vi "ziZoomFFT-SNR.vi"(7 "window properties":cluster{"eq noise BW":dbl, "coherent gain":dbl}={"eq noise BW"=1.0, "coherent gain"=1.0} {"coherent gain" format="%0.2f"; "eq noise BW" format="%0.2f"}, 8 "Order (#)":i32=8, 9 "Timeconstant (s)":dbl format="%#_3p", 10 "Powerspectrum (Vrms^2)":dbl[](array[numeric]), 11 "Freqs (Hz)":dbl[](array[numeric])) -> (0 "Segmentation":cluster{"Freqs (Hz)":dbl[], dbl[]}[](array[cluster]), 1 "Noise BW (Hz)":dbl format="%_3g", 2 "Noise (Vrms^2)":dbl format="%_3g", 3 "Signal BW (Hz)":dbl format="%_3g", 4 "Noise PSD (Vrms/rtHz)":dbl format="%_6p", 5 "Signal (Vrms^2)":dbl format="%_3p", 6 "Peak PSD (Vrms/rtHz)":dbl format="%_6p")   [LabVIEW 2009, in "Zurich Instruments LabOne.lvlib"]
doc: "Calculates:\n\nSNR = \"power in signal band\" / \"power in noise band\"\n\nThe Segmentation output contains an array with:\n\n0: Signal band\n1: Fitted noise\n2: Lower noise band\n3: Upper noise band"
uses:
  <instrlib>/Zurich Instruments LabOne/Zurich Instruments LabOne.lvlib
panel:
  out "Noise Level (Vrms^2)":dbl format="%_6p"
  out "Spectral SNR":dbl format="%_3p"
  out "Segmentation Plot":cluster{"Y":dbl[], "Y":dbl[]}[](graph)
  out "val-trans":dbl[](graph)
  out "Spectral Peak - Noise Separation":dbl format="%_6p"
  out "sorted":dbl[](graph)
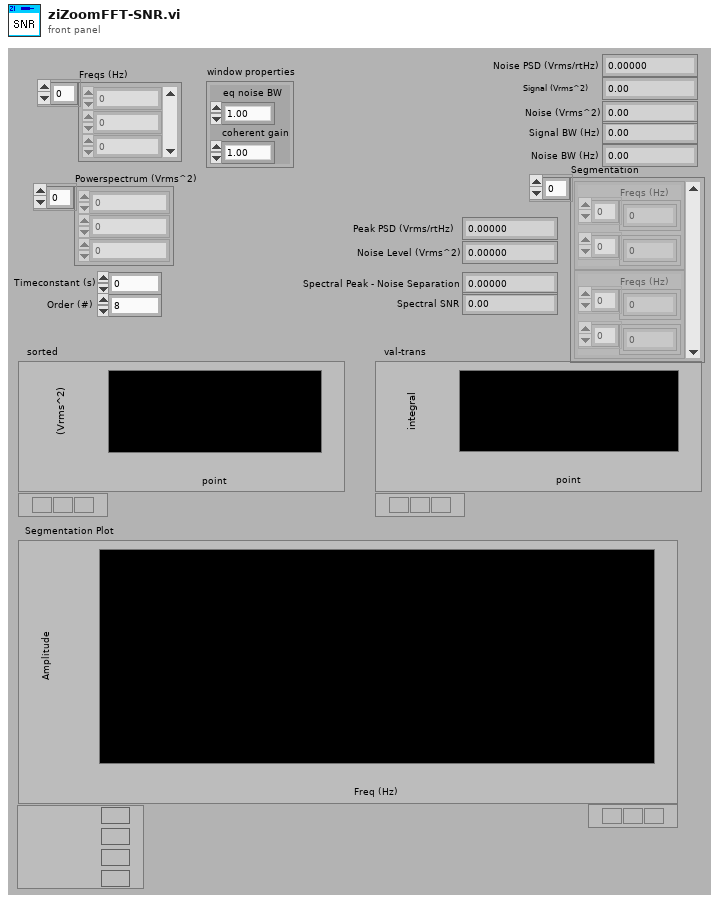
[diagram p1: front panel]
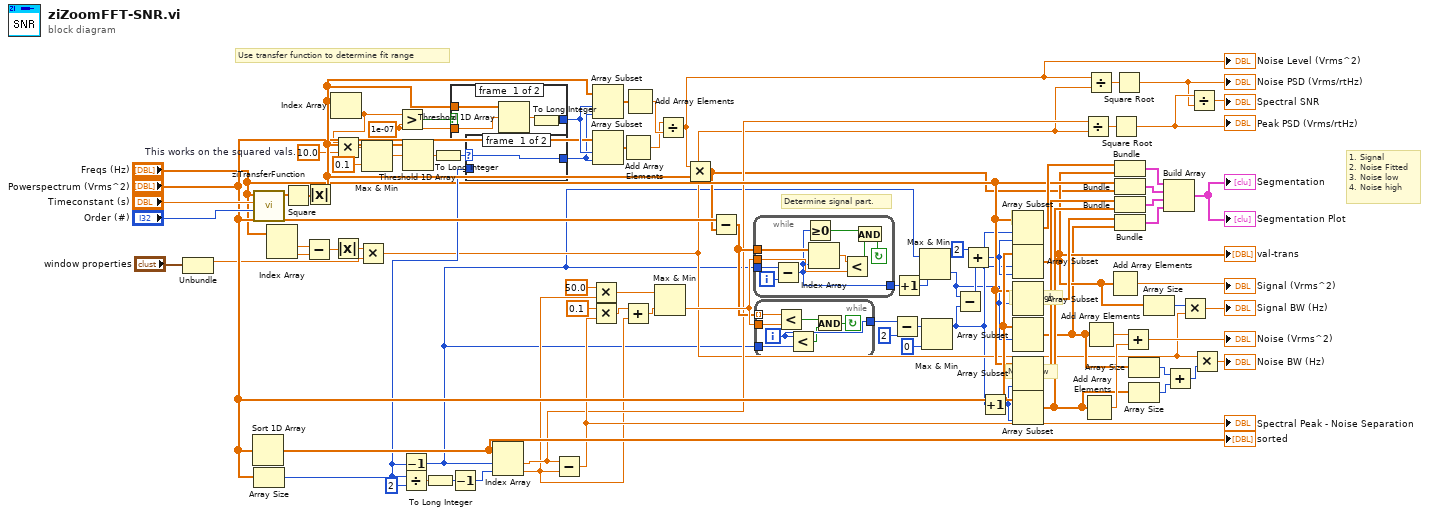
[diagram p0: block diagram]
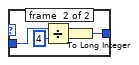
[diagram p2: hidden frame]
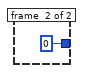
[diagram p3: hidden frame]
diagram:
  w29 = 10.0  # This works on the squared vals.
  w60 = 1e-07 ("y")
  # "Noise Low"
  # "Noise high"
  # "Signal"
  # "1. Signal\n2. Noise Fitted\n3. Noise low\n4. Noise high"
  # "Determine signal part."
  # "Use transfer function to determine fit range"
  n1 = Unbundle("window properties") -> ("eq noise BW"=w42:dbl)  [unwired: 1 out]
  n2 = Sort 1D Array(array="Powerspectrum (Vrms^2)") -> (sorted array=w84:dbl[])
  "sorted" <- w84
  n3 = call <instrlib>:"ziTransferFunction.vi"("Order (#)"="Order (#)", "Timeconstant (s)"="Timeconstant (s)", "Frequencies (Hz)"="Freqs (Hz)") -> ("TransferFunction"=w85:cdb[])  [unwired: 8 in]
  n4 = Array Size(array="Powerspectrum (Vrms^2)") -> (size(s)=w61:i32)
  n5 = Index Array(array="Freqs (Hz)") -> (element #1=w48:dbl, element #2=w47:dbl)  [unwired: 2 in]
  n6 = Square(x=w85) -> (x^2=w83:cdb[])
  n7 = Subtract(x=w48, y=w47) -> (x-y=w46:dbl)
  n8 = Absolute Value(x=w83) -> (abs(x)=w78:dbl[])
  n9 = Index Array(array=w78) -> (element=w30:dbl)  [unwired: 1 in]
  n10 = Multiply(x=w30, y=w29) -> (x*y=w31:dbl)
  n11 = Absolute Value(x=w46) -> (abs(x)=w43:dbl)
  n12 = Multiply(x=w43, y=w42) -> (x*y=w19:dbl)
  n13 = Max & Min(x=w31, y=0.1 ("threshold y")) -> (min(x,y)=w33:dbl)  [unwired: 1 out]
  n14 = Greater?(x=w30, y=w60) -> (0:w80:bool)
  n15 = Decrement(x=w61) -> (x-1=w1:i32)
  n16 = Divide(x=w61, y=2) -> (x/y=w81:dbl)
  n17 = Threshold 1D Array(2:w33, 3:w78) -> (0:w79:dbl)  [unwired: 1 in]
  n18 = To Long Integer(number=w81) -> (32bit integer=w65:i32)
  n19 = To Long Integer(number=w79) -> (32bit integer=w63:i32)
  n20 = Decrement(x=w65) -> (x-1=w64:i32)
  n21 = case shown="True" w80 {
    tunnel: w78 -> [w90 _]
    tunnel: [w88 0] -> w77
    tunnel: w60 -> [w87 _]
    frame #0 {
      n22 = Threshold 1D Array(2:w87, 3:w90) -> (0:w89:dbl)  [unwired: 1 in]
      n23 = To Long Integer(number=w89) -> (32bit integer=w88:i32)
    }
    frame #1 {
    }
  }
  n24 = case shown="0" w63 {
    selector: w63 -> [w92 _]
    tunnel: [w92 w93] -> w62
    tunnel: w61 -> [_ w96]
    frame #0 {
    }
    frame #1 {
      n25 = Divide(x=w96, y=4) -> (x/y=w94:dbl)
      n26 = To Long Integer(number=w94) -> (32bit integer=w93:i32)
    }
  }
  n27 = Index Array(array=w84, index #1=w1, index #2=w64) -> (element #1=w35:dbl, element #2=w8:dbl)
  n28 = Subtract(x=w35, y=w8) -> (x-y=w56:dbl)
  "Spectral Peak - Noise Separation" <- w56
  n29 = Multiply(x=50.0, y=w8) -> (x*y=w58:dbl)
  n30 = Multiply(x=0.1, y=w56) -> (x*y=w55:dbl)
  n31 = Array Subset(array=w78, index=w77, length=w62) -> (w76:dbl[])
  n32 = Array Subset(array="Powerspectrum (Vrms^2)", index=w77, length=w62) -> (w75:dbl[])
  n33 = Add Array Elements(numeric array=w75) -> (sum=w73:dbl)
  n34 = Add(x=w55, y=w8) -> (x+y=w9:dbl)
  n35 = Add Array Elements(numeric array=w76) -> (sum=w74:dbl)
  n36 = Max & Min(x=w58, y=w9) -> (min(x,y)=w59:dbl)  [unwired: 1 out]
  n37 = Divide(x=w73, y=w74) -> (x/y=w41:dbl)
  "Noise Level (Vrms^2)" <- w41
  n38 = Multiply(x=w41, y=w78) -> (x*y=w7:dbl[])
  n39 = Subtract(x="Powerspectrum (Vrms^2)", y=w7) -> (x-y=w54:dbl[])
  n40 = while {
    tunnel: w54 -> [w105]
    tunnel: w59 -> [w102]
    tunnel: w1 -> [w104]
    tunnel: [w97] -> w4
    i -> [w101]
    stop <- w99 continue-if-true
    n41 = Subtract(x=w104, y=w101) -> (x-y=w97:i32)
    n42 = Greater Or Equal To 0?(x=w97) -> (x >= 0?=w98:bool)
    n43 = Index Array(array=w105, index=w97) -> (element=w103:dbl)
    n44 = Less?(x=w103, y=w102) -> (x < y?=w100:bool)
    n45 = And(x=w98, y=w100) -> (x .and. y?=w99:bool)
  }
  n46 = while {
    tunnel: w54 -> [w110] mode=indexing
    tunnel: w59 -> [w112]
    tunnel: [w109] -> w16
    tunnel: w1 -> [w108]
    i -> [w109]
    stop <- w107 continue-if-true
    n47 = Less?(x=w110, y=w112) -> (x < y?=w111:bool)
    n48 = Less?(x=w109, y=w108) -> (x < y?=w106:bool)
    n49 = And(x=w111, y=w106) -> (x .and. y?=w107:bool)
  }
  n50 = Subtract(x=w16, y=2 ("x")) -> (x-y=w15:i32)
  n51 = Increment(x=w4) -> (x+1=w3:i32)
  n52 = Max & Min(x=w1, y=w3) -> (min(x,y)=w2:i32)  [unwired: 1 out]
  n53 = Max & Min(x=w15, y=0 ("x")) -> (max(x,y)=w11:i32)  [unwired: 1 out]
  n54 = Subtract(x=w2, y=w11) -> (x-y=w10:i32)
  n55 = Add(x=2, y=w10) -> (x+y=w12:i32)
  n56 = Increment(x=w11) -> (x+1=w6:i32)
  n57 = Array Subset(array="Freqs (Hz)", index=w11, length=w12) -> (w67:dbl[])
  n58 = Array Subset(array="Powerspectrum (Vrms^2)", index=w11, length=w12) -> (w25:dbl[])
  "val-trans" <- w25
  n59 = Array Subset(array="Freqs (Hz)", index=w2) -> (w66:dbl[])  [unwired: 1 in]
  n60 = Array Subset(array="Powerspectrum (Vrms^2)", index=w2) -> (w24:dbl[])  [unwired: 1 in]
  n61 = Array Subset(array="Freqs (Hz)", length=w6) -> (w68:dbl[])  [unwired: 1 in]
  n62 = Array Subset(array="Powerspectrum (Vrms^2)", length=w6) -> (w26:dbl[])  [unwired: 1 in]
  n63 = Divide(x=w35, y=w19) -> (x/y=w40:dbl)
  n64 = Add Array Elements(numeric array=w26) -> (sum=w34:dbl)
  n65 = Divide(x=w41, y=w19) -> (x/y=w44:dbl)
  n66 = Add Array Elements(numeric array=w24) -> (sum=w36:dbl)
  n67 = Add Array Elements(numeric array=w25) -> (sum=→"Signal (Vrms^2)":dbl)
  n68 = Square Root(x=w40) -> (sqrt(x)=w39:dbl)
  "Peak PSD (Vrms/rtHz)" <- w39
  n69 = Square Root(x=w44) -> (sqrt(x)=w38:dbl)
  "Noise PSD (Vrms/rtHz)" <- w38
  n70 = Bundle(w67, w25) -> (w53:cluster{dbl[], dbl[]})  [unwired: 1 in]
  n71 = Bundle("Freqs (Hz)"="Freqs (Hz)", w7) -> (w52:cluster{"Freqs (Hz)":dbl[], dbl[]})  [unwired: 1 in]
  n72 = Bundle(w68, w26) -> (w51:cluster{dbl[], dbl[]})  [unwired: 1 in]
  n73 = Bundle(w66, w24) -> (w50:cluster{dbl[], dbl[]})  [unwired: 1 in]
  n74 = Add(x=w36, y=w34) -> (x+y=→"Noise (Vrms^2)":dbl)
  n75 = Array Size(array=w24) -> (size(s)=w22:i32)
  n76 = Array Size(array=w26) -> (size(s)=w23:i32)
  n77 = Array Size(array=w25) -> (size(s)=w21:i32)
  n78 = Build Array(w53, w52, w51, w50) -> (→"Segmentation Plot" →"Segmentation":cluster{"Freqs (Hz)":dbl[], dbl[]}[])
  n79 = Add(x=w22, y=w23) -> (x+y=w20:i32)
  n80 = Multiply(x=w21, y=w19) -> (x*y=→"Signal BW (Hz)":dbl)
  n81 = Divide(x=w39, y=w38) -> (x/y=→"Spectral SNR":dbl)
  n82 = Multiply(x=w19, y=w20) -> (x*y=→"Noise BW (Hz)":dbl)
